vi "counterTest.vi"() -> ()   [LabVIEW 2017]
uses:
  <vilib>/DAQmx/read.llb/DAQmx Read (Counter U32 1Chan 1Samp).vi
  <vilib>/DAQmx/read.llb/DAQmx Read (Analog DBL 1Chan 1Samp).vi
  <vilib>/DAQmx/write.llb/DAQmx Write (Digital Bool 1Line 1Point).vi
  <vilib>/DAQmx/write.llb/DAQmx Write (Analog DBL 1Chan 1Samp).vi
  <vilib>/DAQmx/create/channels.llb/DAQmx Create Channel (AO-Voltage-Basic).vi
  <vilib>/DAQmx/create/channels.llb/DAQmx Create Channel (DO-Digital Output).vi
  <vilib>/DAQmx/create/channels.llb/DAQmx Create Channel (AI-Voltage-Basic).vi
  <vilib>/DAQmx/configure/timing.llb/DAQmx Timing (Sample Clock).vi
  globalDevices.vi
  <vilib>/DAQmx/miscellaneous.llb/DAQmx Fill In Error Info.vi
panel:
  in  "stop 4":bool
  in  "data 2":bool
  out "Waveform Chart":dbl(graph)
  out "Waveform Chart 2":dbl(graph)
  in  "stop 3":bool
  in  "stop 2":bool
  out "data":u32
  in  "stop":bool
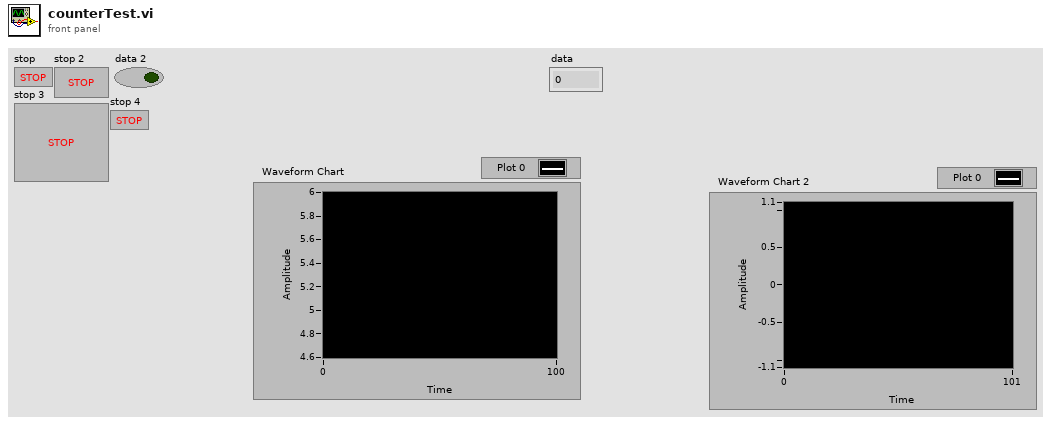
[diagram p1: front panel]
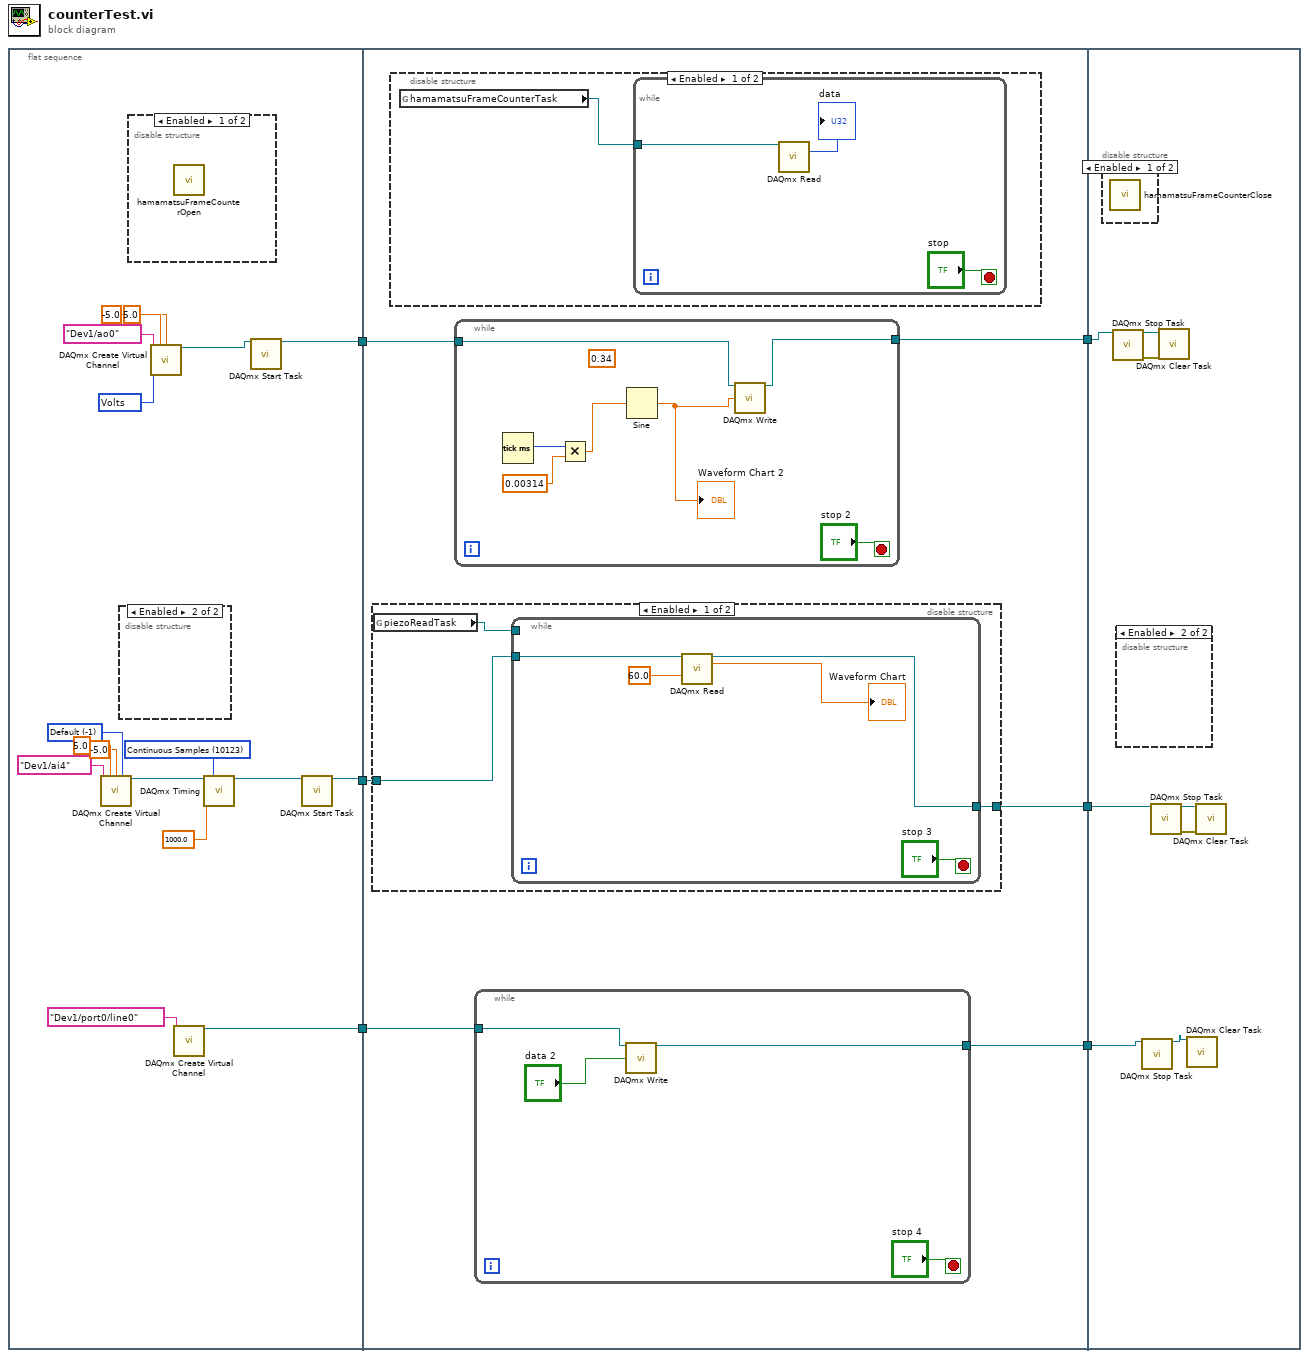
[diagram p0: block diagram]
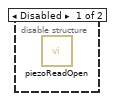
[diagram p2: hidden frame]
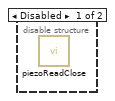
[diagram p6: hidden frame]
diagram:
  n1 = flat-sequence {
    tunnel: [w21] -> w6
    tunnel: [w16] -> w4
    tunnel: [w12] -> w2
    tunnel: w6 -> [w29]
    tunnel: [w28] -> w5
    tunnel: w4 -> [w27]
    tunnel: [w26] -> w3
    tunnel: w2 -> [w25]
    tunnel: [w24] -> w1
    tunnel: w5 -> [w60]
    tunnel: w3 -> [w57]
    tunnel: w1 -> [w55]
    frame #0 {
      w8 = 10123 items=["Finite Samples"=10178, "Continuous Samples"=10123, "Hardware Timed Single Point"=12522] ("sample mode")
      w11 = -1 items=["Default"=-1, "RSE"=10083, "NRSE"=10078, "Differential"=10106, "Pseudodifferential"=12529] ("input terminal configuration")
      w20 = 10348 items=["Volts"=10348, "From Custom Scale"=10065] ("units")
      n2 = call-poly <vilib>:"DAQmx Create Virtual Channel.vi"("maximum value"=5.0, "minimum value"=-5.0, "input terminal configuration"=w11, "physical channels"=tag "Dev1/ai4") -> ("task out"=w10:refnum<k21>)  [unwired: 10 in, 1 out]
      n3 = disable-structure shown="Enabled" {
        frame Disabled {
          n4 = call "piezoReadOpen.vi"() -> ()  [unwired: 6 in]
        }
        frame Enabled {
        }
      }
      n5 = disable-structure shown="Enabled" {
        frame Enabled {
          n6 = call "hamamatsuFrameCounterOpen.vi"() -> ()  [unwired: 12 in]
        }
        frame Disabled {
        }
      }
      n7 = call-poly <vilib>:"DAQmx Create Virtual Channel.vi"("maximum value"=5.0, "minimum value"=-5.0, "physical channels"=tag "Dev1/ao0", "units"=w20) -> ("task out"=w22:refnum<k21>)  [unwired: 10 in, 1 out]
      n8 = call-poly <vilib>:"DAQmx Create Virtual Channel.vi"("lines"=tag "Dev1/port0/line0") -> ("task out"=w16:refnum<k21>)  [unwired: 13 in, 1 out]
      n9 = call-poly <vilib>:"DAQmx Timing.vi"("task/channels in"=w10, "sample mode"=w8, "rate"=1000.0) -> ("task out"=w7:refnum<k21>)  [unwired: 11 in, 1 out]
      n10 = call <vilib>:"DAQmx Start Task.vi"("task/channels in"=w22) -> ("task out"=w21:refnum<k21>)  [unwired: 13 in, 1 out]
      n11 = call <vilib>:"DAQmx Start Task.vi"("task/channels in"=w7) -> ("task out"=w12:refnum<k21>)  [unwired: 13 in, 1 out]
    }
    frame #1 {
      n12 = disable-structure shown="Enabled" {
        disable-tunnel: w25 -> [w36 _]
        disable-tunnel: [w35 _] -> w24
        frame Enabled {
          n13 = global read "globalDevices.vi" "piezoReadTask"() -> (w34:refnum<k21>)
          n14 = while {
            tunnel: w36 -> [w39]
            tunnel: [w37] -> w35
            tunnel: w34 -> [_]
            stop <- "stop 3" stop-if-true
            n15 = call-poly <vilib>:"DAQmx Read.vi"("task/channels in"=w39, "timeout"=60.0) -> ("task out"=w37:refnum<k21>, "data"=→"Waveform Chart":dbl)  [unwired: 11 in, 1 out]
          }
        }
        frame Disabled {
        }
      }
      n16 = disable-structure shown="Enabled" {
        frame Enabled {
          n17 = global read "globalDevices.vi" "hamamatsuFrameCounterTask"() -> (w42:refnum<k21>)
          n18 = while {
            tunnel: w42 -> [w45]
            stop <- "stop" stop-if-true
            n19 = call-poly <vilib>:"DAQmx Read.vi"("task/channels in"=w45) -> ("data"=→"data":u32)  [unwired: 12 in, 2 out]
          }
        }
        frame Disabled {
        }
      }
      n20 = while {
        tunnel: w29 -> [w49]
        tunnel: [w48] -> w28
        stop <- "stop 2" stop-if-true
        (unwired) 0.34 ("data")
        n21 = Tick Count (ms)() -> (millisecond timer value=w52:u32)
        n22 = Multiply(x=w52, y=0.00314) -> (x*y=w50:dbl)
        n23 = Sine(x=w50) -> (sin(x)=w46:dbl)
        "Waveform Chart 2" <- w46
        n24 = call-poly <vilib>:"DAQmx Write.vi"("task/channels in"=w49, "data"=w46) -> ("task out"=w48:refnum<k21>)  [unwired: 11 in, 2 out]
      }
      n25 = while {
        tunnel: w27 -> [w33]
        tunnel: [w31] -> w26
        stop <- "stop 4" stop-if-true
        n26 = call-poly <vilib>:"DAQmx Write.vi"("task/channels in"=w33, "data"="data 2") -> ("task out"=w31:refnum<k21>)  [unwired: 11 in, 2 out]
      }
    }
    frame #2 {
      n27 = disable-structure shown="Enabled" {
        frame Enabled {
          n28 = call "hamamatsuFrameCounterClose.vi"() -> ()  [unwired: 12 in]
        }
        frame Disabled {
        }
      }
      n29 = call <vilib>:"DAQmx Stop Task.vi"("task/channels in"=w60) -> ("task out"=w59:refnum<k21>, "error out"=w58:errorcluster)  [unwired: 13 in]
      n30 = disable-structure shown="Enabled" {
        frame Disabled {
          n31 = call "piezoReadClose.vi"() -> ()  [unwired: 1 in]
        }
        frame Enabled {
        }
      }
      n32 = call <vilib>:"DAQmx Stop Task.vi"("task/channels in"=w57) -> ("task out"=w56:refnum<k21>)  [unwired: 13 in, 1 out]
      n33 = call <vilib>:"DAQmx Stop Task.vi"("task/channels in"=w55) -> ("task out"=w54:refnum<k21>, "error out"=w53:errorcluster)  [unwired: 13 in]
      n34 = call <vilib>:"DAQmx Clear Task.vi"("task in"=w59, "error in"=w58) -> ()  [unwired: 13 in, 1 out]
      n35 = call <vilib>:"DAQmx Clear Task.vi"("task in"=w56) -> ()  [unwired: 14 in, 1 out]
      n36 = call <vilib>:"DAQmx Clear Task.vi"("task in"=w54, "error in"=w53) -> ()  [unwired: 13 in, 1 out]
    }
  }
